vi "Fan&PowerControl.vi"() -> ()   [LabVIEW 2013]
uses:
  <vilib>/MakerHub/LINX/Public/Peripherals/Digital/Digital Write 1 Chan.vi
  <vilib>/MakerHub/LINX/Public/Peripherals/PWM/PWM Set Duty Cycle 1 Chan.vi
  <vilib>/MakerHub/LINX/Public/Peripherals/Digital/Digital Write N Chans.vi
  <vilib>/MakerHub/LINX/Private/Local IO/LinxDigitalWrite.vi
  <vilib>/MakerHub/LINX/Public/Utilities/Check Channel.vi
  <vilib>/MakerHub/LINX/Public/Utilities/Open Serial.vi
  <vilib>/MakerHub/LINX/Private/Utilties/Generate Error.vi
  <vilib>/MakerHub/LINX/Public/Peripherals/PWM/PWM Set Duty Cycle N Chans.vi
  <vilib>/MakerHub/LINX/LMH-LINX.lvlib
panel:
  out "Light PWM Requested":dbl
  in  "Light Dimmer PWM":u8
  in  "LED Brightness":dbl(slide) scale=0.0..10.0
  out "Fan PWM Requested":dbl
  in  "Fan Speed [%]":dbl(knob) scale=0.0..100.0
  in  "Filament Fans PWM":u8
  in  "Relay Switch 4":bool
  in  "Relay Switch 3":bool
  in  "Relay Switch 2":bool
  in  "DO Channel 4":u8
  in  "DO Channel 3":u8
  in  "DO Channel 2":u8
  in  "End Program":bool
  in  "3D Printer Power":bool
  in  "DO Channel 1":u8
  in  "Serial Port":refnum<visa-resource-name>="COM3"
  # "Tevo Tarantula Power and Fan Control"
  # "Relay Controls"
  # "Filament Fan Control"
  # "Light Control"
  # "The LED on the Relay board should turn off when the switch is activated."
  # "Available PWM Pins (Mega 2560):"
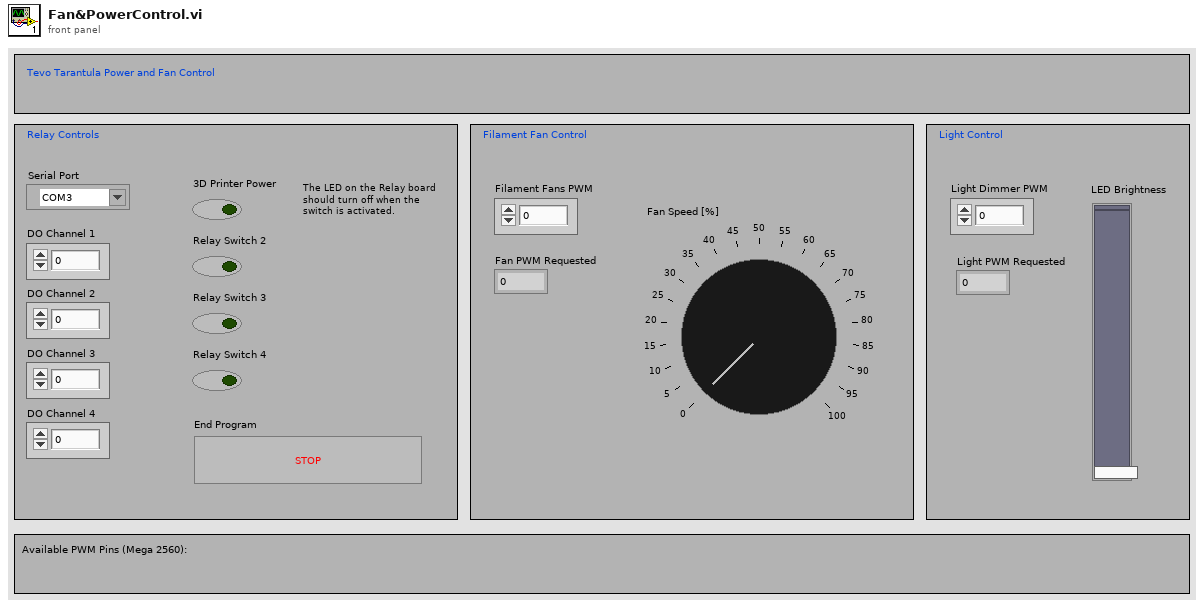
[diagram p1: front panel]
types:
  T1 = typedef "LMH-LINX.lvlib/LINX Ref.ctl" = cluster{"IO":T2, "Interface":T3, "LINX Device Config":T4}
  T2 = typedef "LMH-LINX.lvlib/Platform.ctl" = enum16{"Remote", "Local"}
  T3 = typedef "LMH-LINX.lvlib/Interface.ctl" = enum16{"Serial", "TCP"}
  T4 = typedef "LMH-LINX.lvlib/Device.lvlib/LINX Device Config.ctl" = cluster{"Interface":T3, "COM Port":refnum<visa-resource-name>, "TCP Configuration":T5, "Device Family":u8, "Device ID":u8, "Device Name":string, "TCP Ref":refnum<k5>, "Channels":T6}
  T5 = typedef "LMH-LINX.lvlib/Device.lvlib/TCP Config.ctl" = cluster{"IP Address":string, "Port":u16}
  T6 = typedef "LMH-LINX.lvlib/Channels.ctl" = cluster{"DI":u8[], "DO":u8[], "AI":u8[], "AO":u8[], "PWM":u8[], "QE":u8[], "UART":u8[], "I2C 2":u8[], "SPI":u8[], "CAN":u8[], "Servo":u8[], "AI Ref (V)":dbl, "AI Resolution (Bits)":u8, "AO Ref (V)":dbl, "AO Resolution (Bits)":u8}
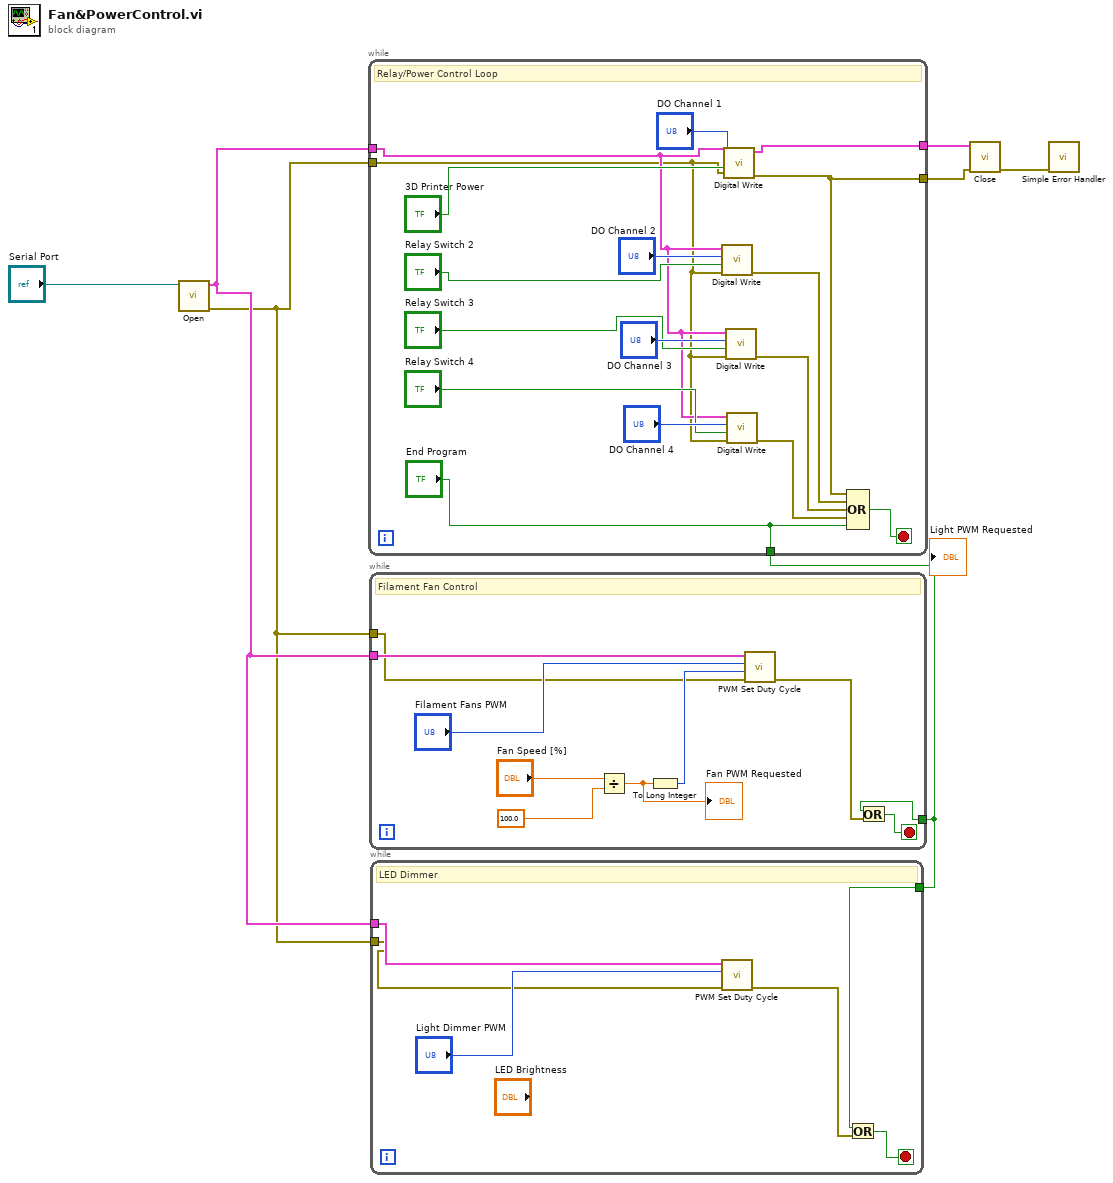
[diagram p0: block diagram]
diagram:
  n1 = call-poly <vilib>:"Open.vi"("Serial Port"="Serial Port") -> ("Error Out"=w1:errorcluster, "LINX Resource"=w2:T1)  [unwired: 8 in, 1 out]
  n2 = while {
    tunnel: w2 -> [w15]
    tunnel: w1 -> [w14]
    tunnel: [w22] -> w6
    tunnel: [w12] -> w5
    tunnel: ["End Program"] -> w3
    stop <- w13 stop-if-true
    # "Relay/Power Control Loop"
    n3 = call-poly <vilib>:"Digital Write.vi"("Error In"=w14, "Output Value"="Relay Switch 2", "DO Channel"="DO Channel 2", "LINX Resource"=w15) -> ("Error Out"=w11:errorcluster)  [unwired: 6 in, 1 out]
    n4 = call-poly <vilib>:"Digital Write.vi"("Error In"=w14, "Output Value"="3D Printer Power", "DO Channel"="DO Channel 1", "LINX Resource"=w15) -> ("Error Out"=w12:errorcluster, "LINX Resource"=w22:T1)  [unwired: 6 in]
    n5 = call-poly <vilib>:"Digital Write.vi"("Error In"=w14, "Output Value"="Relay Switch 3", "DO Channel"="DO Channel 3", "LINX Resource"=w15) -> ("Error Out"=w10:errorcluster)  [unwired: 6 in, 1 out]
    n6 = call-poly <vilib>:"Digital Write.vi"("Error In"=w14, "Output Value"="Relay Switch 4", "DO Channel"="DO Channel 4", "LINX Resource"=w15) -> ("Error Out"=w9:errorcluster)  [unwired: 6 in, 1 out]
    n7 = Compound Arithmetic op=OR(w12, w11, w10, w9, "End Program") -> (w13:bool)
  }
  n8 = while {
    tunnel: w1 -> [w29]
    tunnel: w2 -> [w34]
    tunnel: w3 -> [w26]
    stop <- w28 stop-if-true
    # "Filament Fan Control"
    n9 = Divide(x="Fan Speed [%]", y=100.0) -> (x/y=w25:dbl)
    "Fan PWM Requested" <- w25
    n10 = To Long Integer(number=w25) -> (32bit integer=w30:i32)
    n11 = call-poly <vilib>:"PWM Set Duty Cycle.vi"("Error In"=w29, "Duty Cycle (0-1)"=w30, "PWM Channel"="Filament Fans PWM", "LINX Resource"=w34) -> ("Error Out"=w27:errorcluster)  [unwired: 6 in, 1 out]
    n12 = Or(x=w26, y=w27) -> (x .or. y?=w28:bool)
  }
  n13 = while {
    tunnel: w3 -> [w39]
    tunnel: w2 -> [w36]
    tunnel: w1 -> [w35]
    stop <- w40 stop-if-true
    # "LED Dimmer"
    n14 = call-poly <vilib>:"PWM Set Duty Cycle.vi"("Error In"=w35, "PWM Channel"="Light Dimmer PWM", "LINX Resource"=w36) -> ("Error Out"=w38:errorcluster)  [unwired: 7 in, 1 out]
    n15 = Or(x=w39, y=w38) -> (x .or. y?=w40:bool)
  }
  n16 = call <vilib>:"Close.vi"("Error In"=w5, "LINX Resource"=w6) -> ("Error Out"=w4:errorcluster)  [unwired: 9 in]
  n17 = call <vilib>:"Simple Error Handler.vi"("error in (no error)"=w4) -> ()  [unwired: 4 in, 5 out]
